vi "TxImgSlice.vi"(7 "address":cluster{"address":u32, "port":u16}, 8 "error in":errorcluster, 10 "DataString":string, 11 "Conn":refnum<k16>) -> (0 "error out":errorcluster, 3 "Conn":refnum<k16>)   [LabVIEW 2020]
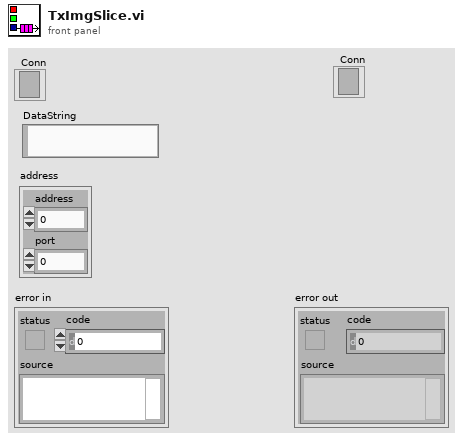
[diagram p1: front panel]
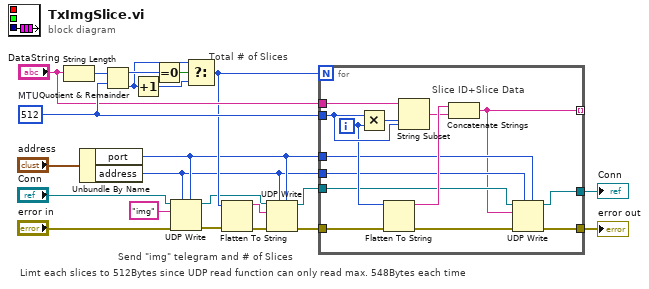
[diagram p0: block diagram]
diagram:
  w19 = 512  # MTU
  # "Limt each slices to 512Bytes since UDP read function can only read max. 548Bytes each time"
  # "Send \"img\" telegram and # of Slices"
  # "Total # of Slices"
  n1 = String Length(string="DataString") -> (length=w22:i32)
  n2 = Unbundle By Name("address") -> ("port"=w7:u16, "address"=w6:u32)
  n3 = Quotient & Remainder(x=w22, y=w19) -> (x-y*floor(x/y)=w17:i32, floor(x/y)=w16:i32)
  n4 = Increment(x=w16) -> (x+1=w20:i32)
  n5 = Equal To 0?(x=w17) -> (x = 0?=w21:bool)
  n6 = UDP Write(address=w6, port or service name=w7, connection ID="Conn", data in="img", 8:"error in") -> (error out=w3:errorcluster, 3:w2:refnum<k16>)  [unwired: 1 in]
  n7 = Select(t=w16, s=w21, f=w20) -> (s? t:f=w9:i32)
  n8 = Flatten To String(anything=w9, error in (no error)=w3) -> (data string=w11:string, error out=w12:errorcluster)  [unwired: 3 out]
  n9 = UDP Write(address=w6, port or service name=w7, connection ID=w2, data in=w11, 8:w12) -> (error out=w13:errorcluster, 3:w10:refnum<k16>)  [unwired: 1 in]
  n10 = for {
    N: w9 -> [_]
    tunnel: w19 -> [w35]
    tunnel: "DataString" -> [w34]
    tunnel: w13 -> [w31]
    tunnel: w10 -> [w29]
    tunnel: [w28] -> w15
    tunnel: [w27] -> w14
    tunnel: w7 -> [w26]
    tunnel: w6 -> [w25]
    tunnel: [w23] -> _ mode=indexing
    i -> [w32]
    # "Slice ID+Slice Data"
    n11 = Multiply(x=w35, y=w32) -> (x*y=w36:i32)
    n12 = Flatten To String(anything=w32, error in (no error)=w31) -> (data string=w33:string, error out=w24:errorcluster)  [unwired: 3 out]
    n13 = String Subset(string=w34, offset (0)=w36, length (rest)=w35) -> (substring=w30:string)
    n14 = Concatenate Strings(w33, w30) -> (w23:string)
    n15 = UDP Write(address=w25, port or service name=w26, connection ID=w29, data in=w23, 8:w24) -> (error out=w28:errorcluster, 3:w27:refnum<k16>)  [unwired: 1 in]
  }
  "error out" <- w15
  "Conn" <- w14
